vi "Begin.vi"(8 "error in (no error)":errorcluster, 11 "GrabberArms in":refnum<class "GrabberArms.lvclass">) -> (0 "error out":errorcluster, 3 "GrabberArms out":refnum<class "GrabberArms.lvclass">)   [LabVIEW 2013, in "GrabberArms.lvclass"]
uses:
  GrabberArms.lvclass
  <vilib>/Rock Robotics/SystemInterfaces/Typedef/FPGA_TypedefSolenoidModule.ctl
  <vilib>/Rock Robotics/WPI/Solenoid/WPI_SolenoidChannel.ctl
  <vilib>/Rock Robotics/SystemInterfaces/DIO/FPGA_DIOChannel.ctl
  System/System.lvclass
  <vilib>/Rock Robotics/WPI/Solenoid/WPI_SolenoidOpenSingle.vi
panel:
  in  "DIO Channel":T1=enum."DIO 8"
  in  "GA Solenoid Channel":T2
  in  "GA Solenoid Module":T3
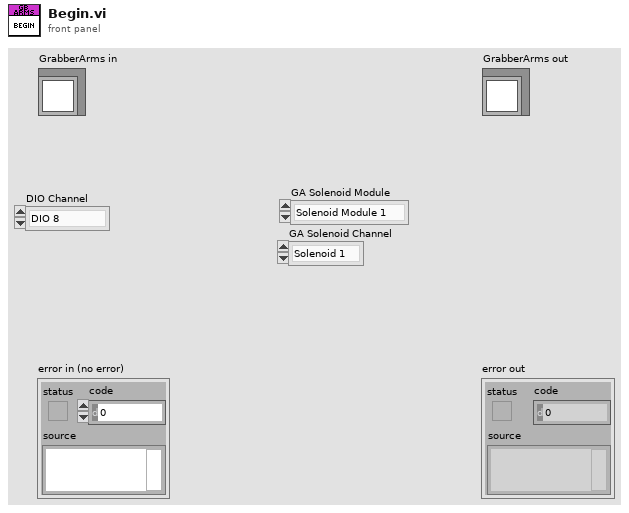
[diagram p1: front panel]
types:
  T1 = typedef "FPGA_DIOChannel.ctl" = enum8{"DIO 1", "DIO 2", "DIO 3", "DIO 4", "DIO 5", "DIO 6", "DIO 7", "DIO 8", "DIO 9", "DIO 10", "DIO 11", "DIO 12", "DIO 13", "DIO 14", "Invalid"}
  T2 = typedef "WPI_SolenoidChannel.ctl" = enum8{"Solenoid 1", "Solenoid 2", "Solenoid 3", "Solenoid 4", "Solenoid 5", "Solenoid 6", "Solenoid 7", "Solenoid 8", "Invalid"}
  T3 = typedef "FPGA_TypedefSolenoidModule.ctl" = enum16{"Solenoid Module 1", "Solenoid Module 2"}
  T4 = typedef "WPI_SolenoidDevRef.ctl" = cluster{"DevStatus":errorcluster, "Solenoid Module":T3, "Forward Solenoid Channel":T2, "Reverse Solenoid Channel":T2}
  T5 = typedef "WPI_DigitalInputDevRef.ctl" = cluster{"DevStatus":errorcluster, "DIO Channel":T1, "Digital Module":T6}
  T6 = typedef "FPGA_TypedefDigitalModule.ctl" = enum16{"Digital Module 1", "Digital Module 2"}
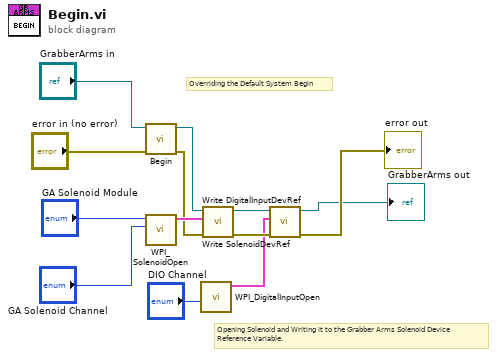
[diagram p0: block diagram]
diagram:
  # "Overriding the Default System Begin"
  # "Opening Solenoid and Writing it to the Grabber Arms Solenoid Device\nReference Variable."
  n1 = call-parent "Begin.vi"("error in (no error)"="error in (no error)", "System in"="GrabberArms in") -> ("error out"=w5:errorcluster, "System out"=w10:refnum<class "GrabberArms.lvclass">)  [unwired: 8 in]
  n2 = call-poly <vilib>:"WPI_SolenoidOpen.vi"("Solenoid Channel"="GA Solenoid Channel", "Solenoid Module (Module 1)"="GA Solenoid Module") -> ("SolenoidDevRef"=w8:T4)  [unwired: 8 in, 1 out]
  n3 = call <vilib>:"WPI_DigitalInputOpen.vi"("DIO Channel"="DIO Channel") -> ("DigitalInputDevRef"=w2:T5)  [unwired: 9 in, 1 out]
  n4 = call-dynamic "Write SolenoidDevRef.vi"("error in (no error)"=w5, "SolenoidDevRef"=w8, "GrabberArms in"=w10) -> ("error out"=→"error out":errorcluster, "GrabberArms out"=w9:refnum<class "GrabberArms.lvclass">)  [unwired: 7 in]
  n5 = call-dynamic "Write DigitalInputDevRef.vi"("DigitalInputDevRef"=w2, "GrabberArms in"=w9) -> ("GrabberArms out"=→"GrabberArms out":refnum<class "GrabberArms.lvclass">)  [unwired: 8 in, 1 out]
